vi "Message Box_Ok_Cancel.vi"(8 "Cancel_buttonName":string="Cancel", 9 "Ok_buttonName":string="OK", 11 "Message":string) -> (3 "True/False":bool)   [LabVIEW 2022 SP3]
panel:
  in  "Cancel Button":bool
  in  "OK Button":bool
  out "txtMessage":string
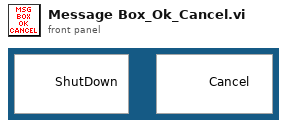
[diagram p1: front panel]
types:
  T1 = enum8{"Enabled", "Disabled", "Disabled and Grayed Out"}
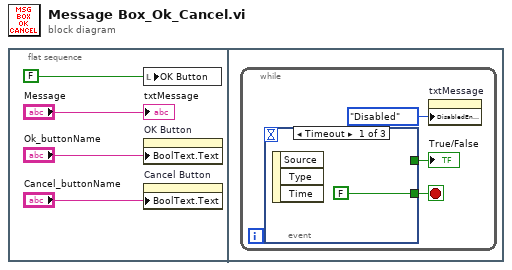
[diagram p0: block diagram]
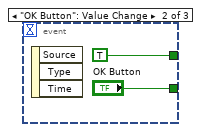
[diagram p2: hidden frame]
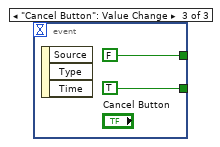
[diagram p3: hidden frame]
diagram:
  n1 = flat-sequence {
    frame #0 {
      n2 = local write "OK Button"(FALSE ("OK Button")) -> ()
      n3 = property on="OK Button" class="Bool (strict)"("BoolText.Text"="Ok_buttonName") -> ()  [unwired: 2 in, 2 out]
      n4 = property on="Cancel Button" class="Bool (strict)"("BoolText.Text"="Cancel_buttonName") -> ()  [unwired: 2 in, 2 out]
      "txtMessage" <- "Message"
    }
    frame #1 {
      n5 = while {
        stop <- w7 stop-if-true
        n6 = event shown="[0] Timeout" {
          selector: _ -> [_ _ _]
          dyn-events: _ -> [_ _ _]
          timeout: _ -> [_ _ _]
          tunnel: [FALSE ("OK Button") "OK Button" TRUE ("OK Button")] -> w7
          tunnel: [_ TRUE ("OK Button") FALSE ("OK Button")] -> w5
          event Timeout {
            n7 = event-data() -> ()  [unwired: 1 in, 3 out]
          }
          event "OK Button": Value Change {
            n8 = event-data() -> ()  [unwired: 1 in, 3 out]
          }
          event "Cancel Button": Value Change {
            n9 = event-data() -> ()  [unwired: 1 in, 3 out]
          }
        }
        "True/False" <- w5
        n10 = property on="txtMessage" class="Str"("DisabledEnum"=T1."Disabled" ("Disabled")) -> ()  [unwired: 2 in, 2 out]
      }
    }
  }
